vi "Execute.vi"(8 "error in (no error)":errorcluster, 9 "Workspace":T1, 10 "Cluster":T2={"I-O.lvclass"=refnum, "Gantry"=refnum, "Dispenser"="COM1"}, 11 "Pick and Place in":refnum<class "Pick and Place.lvclass">) -> (0 "error out":errorcluster, 2 "Control Out":T2={"I-O.lvclass"=refnum, "Gantry"=refnum, "Dispenser"="COM1"}, 3 "Pick and Place out":refnum<class "Pick and Place.lvclass">)   [LabVIEW 2018, in "Pick and Place.lvclass"]
uses:
  Pick and Place.lvclass
  Controller/Controllers.ctl
  Controller/I-O/I-O.lvclass
  C:/Program Files (x86)/Aerotech/A3200/LabVIEW/2010/Bin/Aerotech.A3200.dll
  Program Files (x86)/Aerotech/A3200/LabVIEW/2010/Bin/Aerotech.A3200.dll
  Workspace/Workspace.ctl
  Pick and Place.lvclass/Pick and Place.ctl
  Controller/Motion/Motion.lvclass
  Controller/Motion/A3200/A3200.lvclass
  Controller/Controller.lvclass
  Workspace/Fixture.lvclass
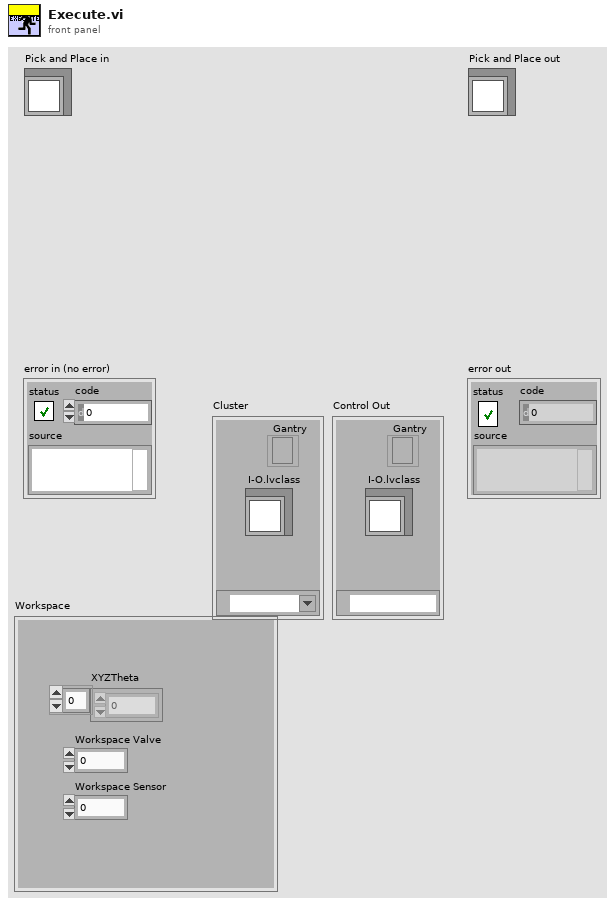
[diagram p1: front panel]
types:
  T1 = typedef "Fixture.lvclass/Workspace.ctl" = cluster{"XYZTheta":dbl[], "Workspace Valve":i32, "Workspace Sensor":i32}
  T2 = typedef "Controller.lvclass/Controllers.ctl" = cluster{"I-O.lvclass":refnum<class "I-O.lvclass">, "Gantry":refnum<k24>, "Dispenser":refnum<visa-resource-name>}
  T3 = typedef "Pick and Place.lvclass/Pick and Place Type.ctl" = enum16{"Primary Pick Up", "Secondary Pick Up", "Put Down All", "Pick Up All", "Put Down Secondary"}
  T4 = typedef "I-O.lvclass/Pin Map.ctl" = cluster{"Region Valves":i32[], "Extra Valves":dbl[][][], "Tool Primary Valve":i32, "Tool Secondary Valve":i32, "Region Sensors":i32[], "Extra Sensors":dbl[][][], "Tool Primary Sensor":dbl, "Tool Secondary Sensor":dbl, "Compression Sensor":dbl, "5V":i32, "Dispenser Sensor":dbl}
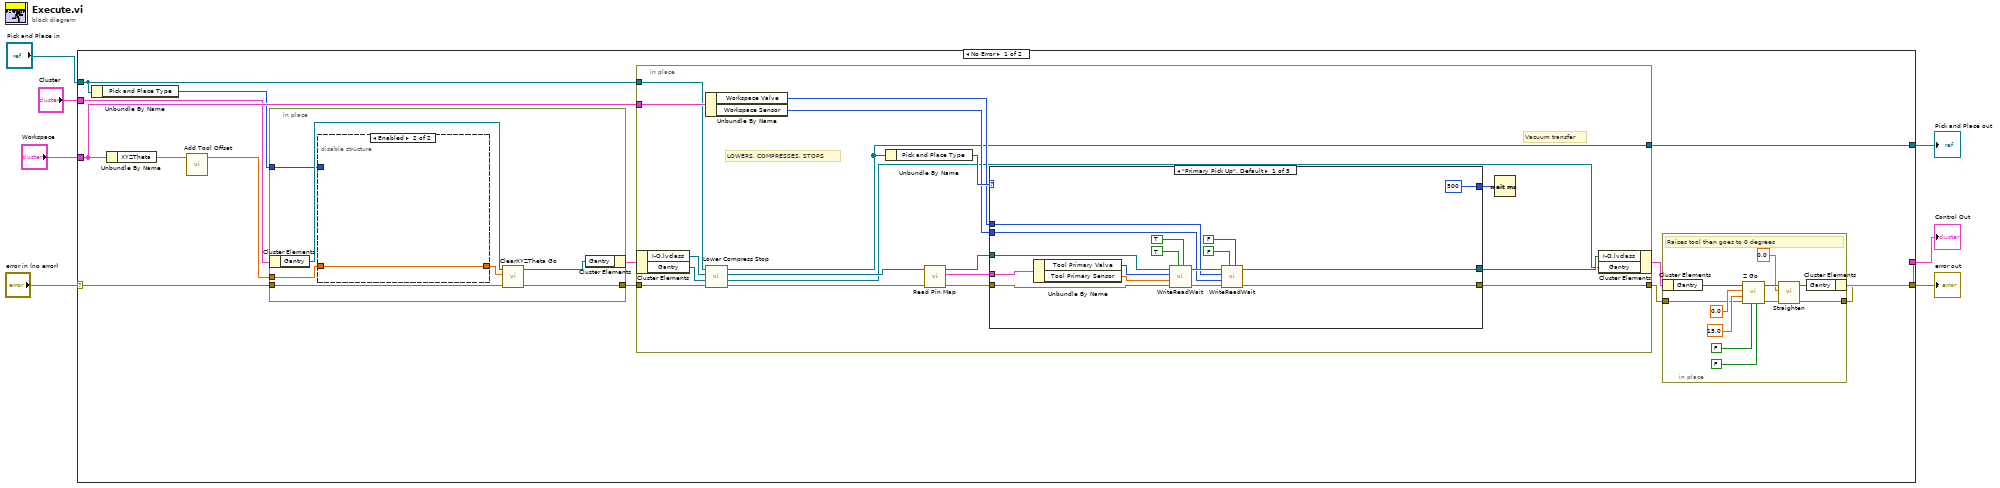
[diagram p0: block diagram]
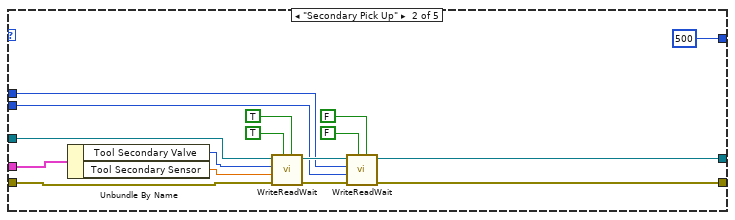
[diagram p2: hidden frame]
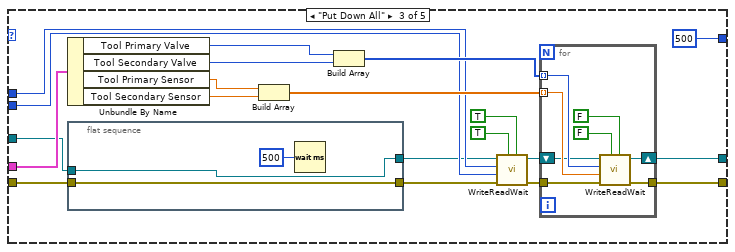
[diagram p3: hidden frame]
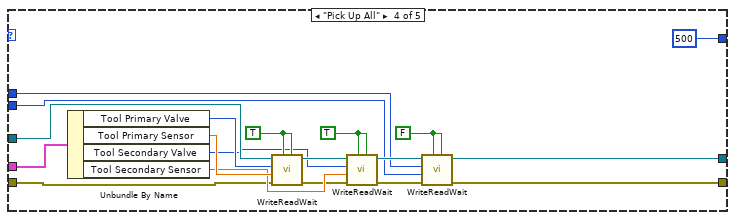
[diagram p4: hidden frame]
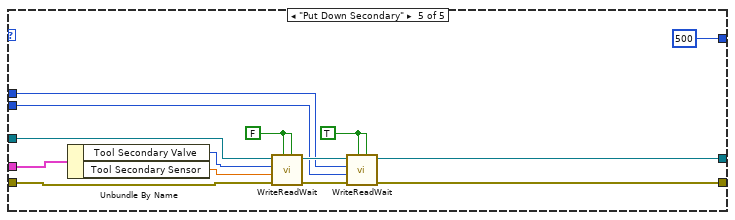
[diagram p5: hidden frame]
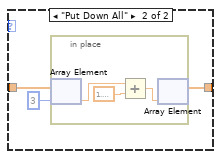
[diagram p7: hidden frame]
diagram:
  n1 = case shown="No Error" "error in (no error)" {
    selector: "error in (no error)" -> [w15 w166]
    tunnel: "Cluster" -> [w19 w167]
    tunnel: "Workspace" -> [w20 _]
    tunnel: [w14 w166] -> w1
    tunnel: [w18 w167] -> w2
    tunnel: "Pick and Place in" -> [w9 w165]
    tunnel: [w17 w165] -> w6
    frame No Error {
      n2 = Unbundle By Name(w9) -> ("Pick and Place Type"=w8:T3)
      n3 = Unbundle By Name(w20) -> ("XYZTheta"=w12:dbl[])
      n4 = call "Add Tool Offset.vi"("XYZTheta"=w12) -> ("Array"=w16:dbl[])  [unwired: 10 in]
      n5 = in-place {
        in-place-border: w16 -> [w148]
        in-place-border: w15 -> [w150]
        in-place-border: [w151] -> w11
        in-place-border: w8 -> [w149]
        n6 = in-place-cluster #1(w19) -> ("Gantry"=w153:refnum<k24>)
        n7 = disable-structure shown="Enabled" {
          disable-tunnel: w149 -> [w156 _]
          disable-tunnel: w148 -> [w155 w164]
          disable-tunnel: [w154 w164] -> w147
          frame Disabled {
            n8 = case shown="\"Primary Pick Up\", Default" w156 {
              tunnel: w155 -> [w157 w160]
              tunnel: [w157 w158] -> w154
              frame "Primary Pick Up", Default {
              }
              frame "Put Down All" {
                n9 = in-place {
                  n10 = in-place-array #2(w160, 3) -> (w163:dbl)
                  n11 = Add(x=w163, y=1.5707963267948966) -> (x+y=w161:dbl)
                  n12 = in-place-array #2(w161) -> (w158:dbl[])  [unwired: 1 out]
                }
              }
            }
          }
          frame Enabled {
          }
        }
        n13 = call "ClearXYZTheta Go.vi"("error in (no error)"=w150, "XYZTheta In"=w147, "Gantry In"=w153) -> ("error out"=w151:errorcluster, "Gantry Out"=w152:refnum<k24>)  [unwired: 6 in, 1 out]
        n14 = in-place-cluster #1("Gantry"=w152) -> (w21:T2)
      }
      n15 = in-place {
        in-place-border: w20 -> [w50]
        in-place-border: w9 -> [w40]
        in-place-border: [w39] -> w17
        in-place-border: w11 -> [w34]
        in-place-border: [w33] -> w10
        # "Vacuum transfer"
        # "LOWERS, COMPRESSES, STOPS"
        n16 = in-place-cluster #3(w21) -> ("I-O.lvclass"=w43:refnum<class "I-O.lvclass">, "Gantry"=w38:refnum<k24>)
        n17 = Unbundle By Name(w50) -> ("Workspace Valve"=w48:i32, "Workspace Sensor"=w47:i32)
        n18 = call "Lower Compress Stop.vi"("error in (no error)"=w34, "Gantry In"=w38, "I-O.lvclass"=w43, "Pick and Place in"=w40) -> ("error out"=w36:errorcluster, "Gantry Out"=w37:refnum<k24>, "I-O out"=w41:refnum<class "I-O.lvclass">, "Pick and Place Out"=w39:refnum<class "Pick and Place.lvclass">)  [unwired: 4 in]
        n19 = Unbundle By Name(w39) -> ("Pick and Place Type"=w49:T3)
        n20 = call-dynamic "Read Pin Map.vi"("error in (no error)"=w36, "I-O in"=w41) -> ("error out"=w35:errorcluster, "Pin Map 2"=w45:T4, "I-O out"=w44:refnum<class "I-O.lvclass">)  [unwired: 7 in]
        n21 = case shown="\"Primary Pick Up\", Default" w49 {
          tunnel: w48 -> [w63 w74 w92 w122 w140]
          tunnel: w47 -> [w62 w73 w91 w121 w139]
          tunnel: [w57 w72 w96 w119 w137] -> w42
          tunnel: [u32 500 ("milliseconds to wait") 500 500 u32 500 ("milliseconds to wait") u32 500 ("milliseconds to wait")] -> w46
          tunnel: w44 -> [w56 w71 w87 w131 w145]
          tunnel: w45 -> [w55 w70 w90 w132 w146]
          tunnel: w35 -> [w53 w69 w84 w117 w135]
          tunnel: [w51 w67 w83 w114 w133] -> w33
          frame "Primary Pick Up", Default {
            n22 = Unbundle By Name(w55) -> ("Tool Primary Valve"=w54:i32, "Tool Primary Sensor"=w65:dbl)
            n23 = call "WriteReadWait.vi"("Read Value"=TRUE, "Write Value"=TRUE, "error in (no error)"=w53, "Read"=w65, "Write"=w54, "I-O in"=w56) -> ("error out"=w52:errorcluster, "I-O out"=w64:refnum<class "I-O.lvclass">)  [unwired: 4 in]
            n24 = call "WriteReadWait.vi"("Read Value"=FALSE ("Write Value"), "Write Value"=FALSE ("Read Value"), "error in (no error)"=w52, "Read"=w62, "Write"=w63, "I-O in"=w64) -> ("error out"=w51:errorcluster, "I-O out"=w57:refnum<class "I-O.lvclass">)  [unwired: 4 in]
          }
          frame "Secondary Pick Up" {
            n25 = Unbundle By Name(w70) -> ("Tool Secondary Valve"=w76:i32, "Tool Secondary Sensor"=w75:dbl)
            n26 = call "WriteReadWait.vi"("Read Value"=TRUE, "Write Value"=TRUE, "error in (no error)"=w69, "Read"=w75, "Write"=w76, "I-O in"=w71) -> ("error out"=w68:errorcluster, "I-O out"=w81:refnum<class "I-O.lvclass">)  [unwired: 4 in]
            n27 = call "WriteReadWait.vi"("Read Value"=FALSE ("Write Value"), "Write Value"=FALSE ("Read Value"), "error in (no error)"=w68, "Read"=w73, "Write"=w74, "I-O in"=w81) -> ("error out"=w67:errorcluster, "I-O out"=w72:refnum<class "I-O.lvclass">)  [unwired: 4 in]
          }
          frame "Put Down All" {
            n28 = Unbundle By Name(w90) -> ("Tool Primary Valve"=w97:i32, "Tool Secondary Valve"=w98:i32, "Tool Primary Sensor"=w99:dbl, "Tool Secondary Sensor"=w100:dbl)
            n29 = flat-sequence {
              tunnel: [w104] -> w88
              tunnel: w87 -> [w104]
              tunnel: [w103] -> w85
              tunnel: w84 -> [w103]
              frame #0 {
                # "Delay After Placing"
                n30 = Wait (ms)(milliseconds to wait=u32 500) -> ()  [unwired: 1 out]
              }
            }
            n31 = Build Array(w99, w100) -> (w102:dbl[])
            n32 = Build Array(w97, w98) -> (w101:i32[])
            n33 = call "WriteReadWait.vi"("Read Value"=TRUE, "Write Value"=TRUE, "error in (no error)"=w85, "Read"=w91, "Write"=w92, "I-O in"=w88) -> ("error out"=w86:errorcluster, "I-O out"=w89:refnum<class "I-O.lvclass">)  [unwired: 4 in]
            n34 = for {
              shift-right: [w108] -> w96
              shift-left: w89 -> [w109]
              tunnel: w101 -> [w111] mode=indexing
              tunnel: w102 -> [w110] mode=indexing
              tunnel: w86 -> [w107]
              tunnel: [w106] -> w83
              n35 = call "WriteReadWait.vi"("Read Value"=FALSE ("Write Value"), "Write Value"=FALSE ("Read Value"), "error in (no error)"=w107, "Read"=w110, "Write"=w111, "I-O in"=w109) -> ("error out"=w106:errorcluster, "I-O out"=w108:refnum<class "I-O.lvclass">)  [unwired: 4 in]
            }
          }
          frame "Pick Up All" {
            w120 = FALSE ("Read Value")
            w124 = TRUE ("Write Value")
            w130 = TRUE ("Write Value")
            n36 = Unbundle By Name(w132) -> ("Tool Primary Valve"=w129:i32, "Tool Primary Sensor"=w128:dbl, "Tool Secondary Valve"=w126:i32, "Tool Secondary Sensor"=w125:dbl)
            n37 = call "WriteReadWait.vi"("Read Value"=w130, "Write Value"=w130, "error in (no error)"=w117, "Read"=w128, "Write"=w129, "I-O in"=w131) -> ("error out"=w116:errorcluster, "I-O out"=w127:refnum<class "I-O.lvclass">)  [unwired: 4 in]
            n38 = call "WriteReadWait.vi"("Read Value"=w124, "Write Value"=w124, "error in (no error)"=w116, "Read"=w125, "Write"=w126, "I-O in"=w127) -> ("error out"=w115:errorcluster, "I-O out"=w123:refnum<class "I-O.lvclass">)  [unwired: 4 in]
            n39 = call "WriteReadWait.vi"("Read Value"=w120, "Write Value"=w120, "error in (no error)"=w115, "Read"=w121, "Write"=w122, "I-O in"=w123) -> ("error out"=w114:errorcluster, "I-O out"=w119:refnum<class "I-O.lvclass">)  [unwired: 4 in]
          }
          frame "Put Down Secondary" {
            w138 = TRUE ("Read Value")
            w142 = FALSE ("Write Value")
            n40 = Unbundle By Name(w146) -> ("Tool Secondary Valve"=w144:i32, "Tool Secondary Sensor"=w143:dbl)
            n41 = call "WriteReadWait.vi"("Read Value"=w142, "Write Value"=w142, "error in (no error)"=w135, "Read"=w143, "Write"=w144, "I-O in"=w145) -> ("error out"=w134:errorcluster, "I-O out"=w141:refnum<class "I-O.lvclass">)  [unwired: 4 in]
            n42 = call "WriteReadWait.vi"("Read Value"=w138, "Write Value"=w138, "error in (no error)"=w134, "Read"=w139, "Write"=w140, "I-O in"=w141) -> ("error out"=w133:errorcluster, "I-O out"=w137:refnum<class "I-O.lvclass">)  [unwired: 4 in]
          }
        }
        n43 = Wait (ms)(milliseconds to wait=w46) -> ()  [unwired: 1 out]
        n44 = in-place-cluster #3("I-O.lvclass"=w42, "Gantry"=w37) -> (w13:T2)
      }
      n45 = in-place {
        in-place-border: [w24] -> w14
        in-place-border: w10 -> [w30]
        # "Raises tool then goes to 0 degrees"
        n46 = in-place-cluster #4(w13) -> ("Gantry"=w27:refnum<k24>)
        n47 = call "Z Go.vi"("Increment"=FALSE, "Return Immediately"=FALSE ("Increment"), "error in (no error)"=w30, "Speed In"=15.0 ("speed"), "Position In"=0.0 ("position"), "Gantry In"=w27) -> ("error out"=w25:errorcluster, "Gantry Out"=w29:refnum<k24>)  [unwired: 2 in, 2 out]
        n48 = call "Straighten.vi"("error in (no error)"=w25, "Angle (rad)"=0.0, "Gantry In"=w29) -> ("error out"=w24:errorcluster, "Gantry Out"=w28:refnum<k24>)  [unwired: 7 in]
        n49 = in-place-cluster #4("Gantry"=w28) -> (w18:T2)
      }
    }
    frame Error {
    }
  }
  "error out" <- w1
  "Pick and Place out" <- w6
  "Control Out" <- w2
